vi "wmf_list_modes.vi"(8 "error in (no error)":errorcluster, 11 "camera_name":string) -> (0 "error out":errorcluster, 3 "Modes":T1(array[cluster]))   [LabVIEW 2023, in "Vision.lvlib"]
uses:
  Vision.lvlib
  camera mode.ctl
  bin/Camera.dll
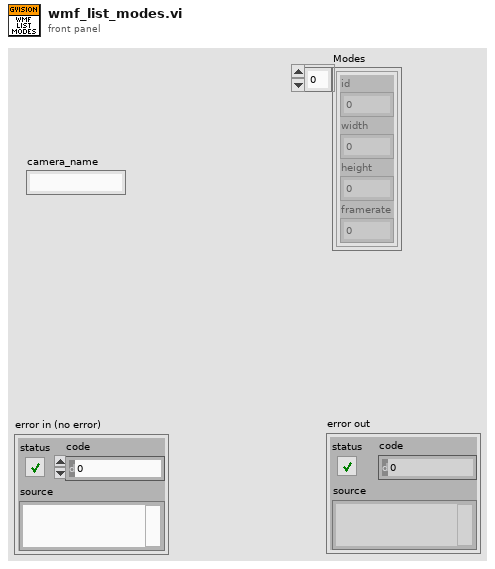
[diagram p1: front panel]
types:
  T1 = cluster{"id":i32, "width":i32, "height":i32, "framerate":sgl}[]
  T2 = typedef "camera mode.ctl" = cluster{"id":i32, "width":i32, "height":i32, "framerate":sgl}
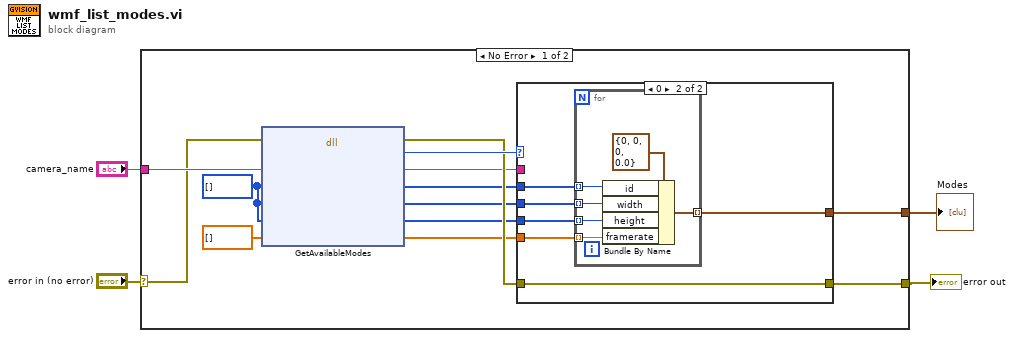
[diagram p0: block diagram]
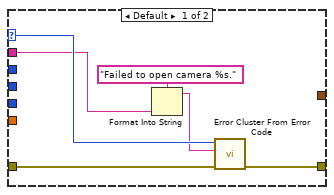
[diagram p2: hidden frame]
diagram:
  n1 = case shown="No Error" "error in (no error)" {
    selector: "error in (no error)" -> [w7 w36]
    tunnel: [w15 w36] -> w2
    tunnel: "camera_name" -> [w14 _]
    tunnel: [w8 _] -> w1
    frame No Error {
      w6 = i32[] [] ("ids")
      n2 = dll-call lib="C:/Users/cfangmeier3/Desktop/nebraska-silicon-lab/pixel-gantry-control/Gantry/Shared Components/bin/Camera.dll" fn="GetAvailableModes"(error in=w7, "cam_name"=w14, "ids"=w6, "widths"=w6, "heights"=w6, "framerates"=sgl[] []) -> (error out=w16:errorcluster, "return type"=w17:i32, "cam_name"=w13:string, "ids"=w12:i32[], "widths"=w11:i32[], "heights"=w10:i32[], "framerates"=w9:sgl[])  [unwired: 2 in, 1 out]
      n3 = case shown="0" w17 {
        selector: w17 -> [w21 _]
        tunnel: w16 -> [w23 w29]
        tunnel: [w22 w29] -> w15
        tunnel: w13 -> [w19 _]
        tunnel: w12 -> [_ w28]
        tunnel: w11 -> [_ w27]
        tunnel: w10 -> [_ w26]
        tunnel: w9 -> [_ w25]
        tunnel: [_ w24] -> w8
        frame Default {
          n4 = Format Into String(format string="Failed to open camera %s." ("error message (\"\")"), w19) -> (resulting string=w18:string)  [unwired: 2 in, 1 out]
          n5 = call <vilib>:"Error Cluster From Error Code.vi"("error in (no error)"=w23, "error message (\"\")"=w18, "error code (0)"=w21) -> ("error out"=w22:errorcluster)  [unwired: 6 in]
        }
        frame 0 {
          n6 = for {
            tunnel: w28 -> [w34] mode=indexing
            tunnel: w27 -> [w33] mode=indexing
            tunnel: w26 -> [w32] mode=indexing
            tunnel: w25 -> [w31] mode=indexing
            tunnel: [w30] -> w24 mode=indexing
            n7 = Bundle By Name(cluster=T2 {"id"=0, "width"=0, "height"=0, "framerate"=0.0}, "id"=w34, "width"=w33, "height"=w32, "framerate"=w31) -> (w30:T2)
          }
        }
      }
    }
    frame Error {
    }
  }
  "error out" <- w2
  "Modes" <- w1
